vi "example batch waitall.vi"() -> ()   [LabVIEW 2013]
uses:
  result/result.lvclass
  standard action/wait action/wait action.lvclass
  standard tasks/batch task/reporting type.ctl
  result/result.lvclass/result.ctl
  result/get data.vi
  result/get error.vi
  result/get generating action.vi
  result/get owning task.vi
  result/get subresults.vi
  dispatcher/thread pool.lvclass
  standard reporters/event reporter/event reporter.lvclass
  standard tasks/batch task/batch task.lvclass
panel:
  out "owning task":string
  out "generating action":string
  out "error":errorcluster
  out "data":variant
  out "accessors:subresults":refnum<class "result.lvclass">[][](array[class])
  out "owning task":string[](array[string])
  out "actions":string[](array[string])
  out "Array 2":errorcluster[](array[cluster])
  out "Array":variant[](array[variant])
  out "Time":u32
  out "result":refnum<class "result.lvclass">
  out "error out":errorcluster
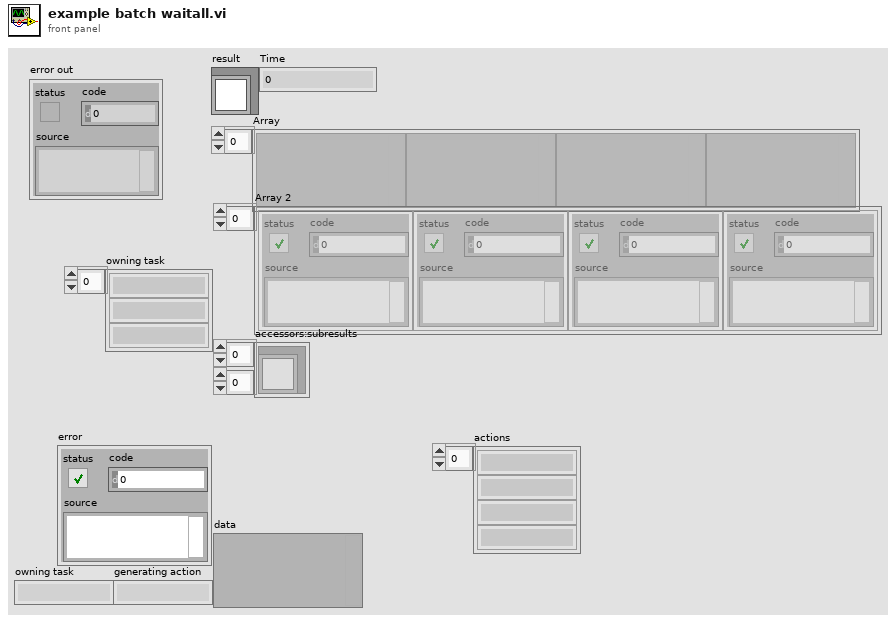
[diagram p1: front panel]
types:
  T1 = typedef "batch task.lvclass/reporting type.ctl" = enum16{"return immediately", "wait on all"}
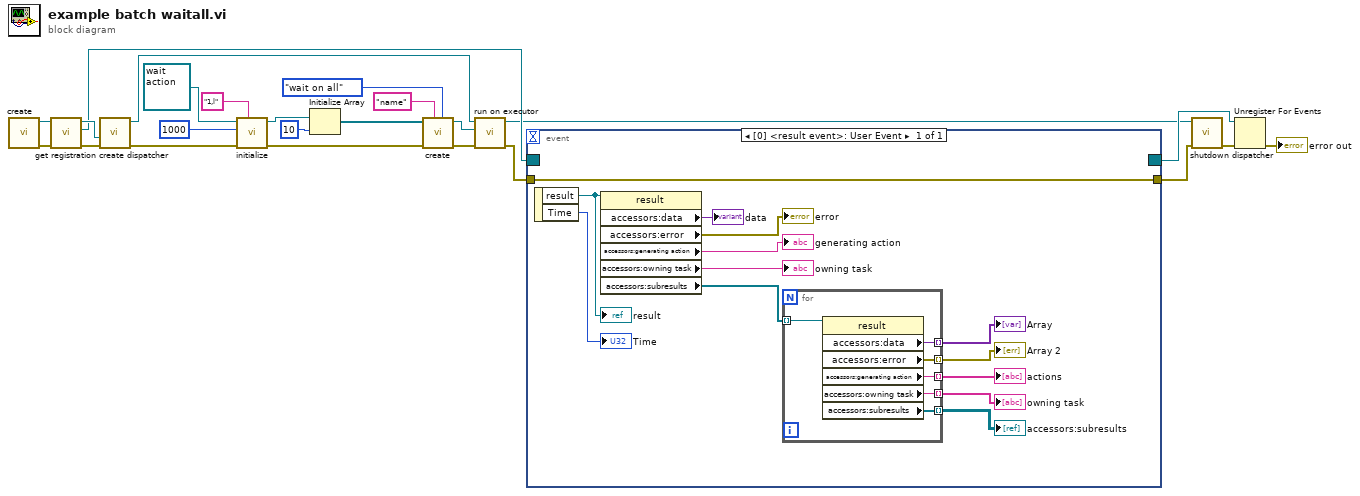
[diagram p0: block diagram]
diagram:
  n1 = call "create.vi"() -> ("error out"=w18:errorcluster, "event reporter out"=w19:refnum<class "event reporter.lvclass">)  [unwired: 10 in]
  n2 = call "get registration.vi"("error in"=w18, "event reporter in"=w19) -> ("error out"=w16:errorcluster, "result registration"=w15:refnum<event-registration>, "event reporter out"=w17:refnum<class "event reporter.lvclass">)  [unwired: 7 in]
  n3 = call "create dispatcher.vi"("error in"=w16, "default reporter"=w17) -> ("error out"=w21:errorcluster, "dispatcher"=w23:refnum<data-value>)  [unwired: 8 in]
  n4 = call-dynamic "initialize.vi"("action name"="1,l", "error in"=w21, "parameters"=1000, "action in"=refnum<class "wait action.lvclass"> refnum ("wait action.lvclass")) -> ("error out"=w6:errorcluster, "action out"=w8:refnum<class "wait action.lvclass">)  [unwired: 6 in]
  n5 = Initialize Array(w8, 10 ("dimension size")) -> (w4:refnum<class "wait action.lvclass">[])
  n6 = call "create.vi"("reporting type"=reporting_type."wait on all", "ID"="name", "actions"=w4) -> ("batch task out"=w3:refnum<class "batch task.lvclass">)  [unwired: 8 in]
  n7 = call "run on executor.vi"("error in"=w6, "task"=w3, "dispatcher"=w23) -> ("error out"=w9:errorcluster, "dispatcher out"=w13:refnum<data-value>)  [unwired: 7 in]
  n8 = event shown="[0] <result event>: User Event" {
    selector: w15 -> [_]
    dyn-events: [_] -> w14
    timeout: _ -> [_]
    tunnel: [w35] -> w10
    tunnel: w9 -> [w35]
    event User Event {
      n9 = event-data() -> ("result"=w34:refnum<class "result.lvclass">, "Time"=→"Time":u32)  [unwired: 1 in]
      "result" <- w34
      n10 = property class="result"(reference=w34) -> ("accessors:data"=→"data":variant, "accessors:error"=→"error":errorcluster, "accessors:generating action"=→"generating action":string, "accessors:owning task"=→"owning task":string, "accessors:subresults"=w33:refnum<class "result.lvclass">[])  [unwired: 1 in, 2 out]
      n11 = for {
        tunnel: w33 -> [w42] mode=indexing
        tunnel: [w41] -> w32 mode=indexing
        tunnel: [w40] -> w31 mode=indexing
        tunnel: [w39] -> w30 mode=indexing
        tunnel: [w38] -> w29 mode=indexing
        tunnel: [w37] -> w28 mode=indexing
        n12 = property class="result"(reference=w42) -> ("accessors:data"=w41:variant, "accessors:error"=w40:errorcluster, "accessors:generating action"=w39:string, "accessors:owning task"=w38:string, "accessors:subresults"=w37:refnum<class "result.lvclass">[])  [unwired: 1 in, 2 out]
      }
      "Array" <- w32
      "Array 2" <- w31
      "actions" <- w30
      "owning task" <- w29
      "accessors:subresults" <- w28
    }
  }
  n13 = call "shutdown dispatcher.vi"("error in"=w10, "dispatcher"=w13) -> ("error out"=w12:errorcluster)  [unwired: 9 in]
  n14 = Unregister For Events(event registration refnum=w14, error in=w12) -> (error out=→"error out":errorcluster)
